vi "M5StackDAC2.vi"() -> ()   [LabVIEW 2024]
uses:
  Driver/Public/Digital Pull Direction.ctl
  4d20a38f-85d9-49a3-8b57-4ea18b2081fb.vi
  31698fb6-f1eb-4e5e-bade-b2e1298fca87.vi
  Driver/CTIPicoVISA.lvlib
panel:
  out "error out":errorcluster
  out "appended array":u8[](array[numeric])=[2, 208, 7, 7, 209] format="%.0x"
  in  "V1":u16(slide)=2001 scale=0.0..32767.0
  in  "V0":u16(slide)=2000 scale=0.0..32767.0
  in  "Grove Connector":enum16{"I2C0", "I2C1"}(ring)
  in  "VISA resource name in":refnum<visa-resource-name>="COM19"
  out "Identity":T1
  # "https://docs.m5stack.com/en/unit/Unit-DAC2"
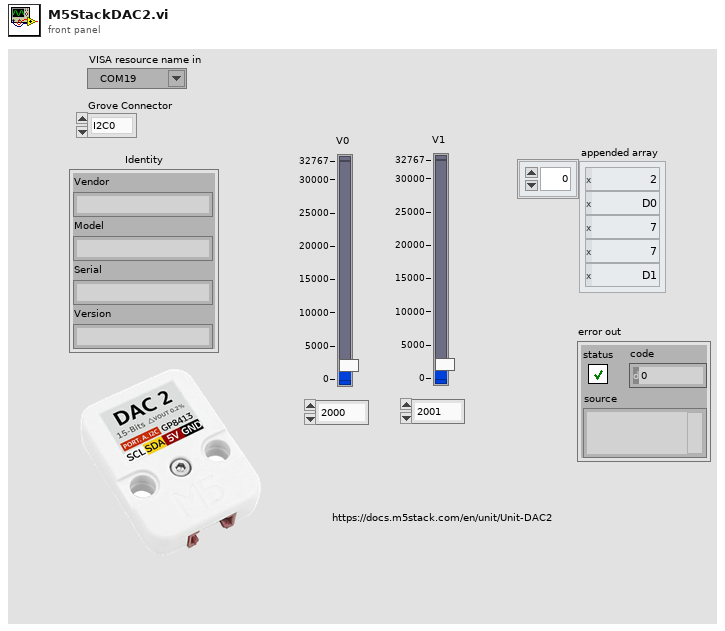
[diagram p1: front panel]
types:
  T1 = cluster{"Vendor":string, "Model":string, "Serial":string, "Version":string}
  T2 = typedef "CTIPicoVISA.lvlib/Digital Pull Direction.ctl" = enum16{"None", "Up", "Down", "Both"}
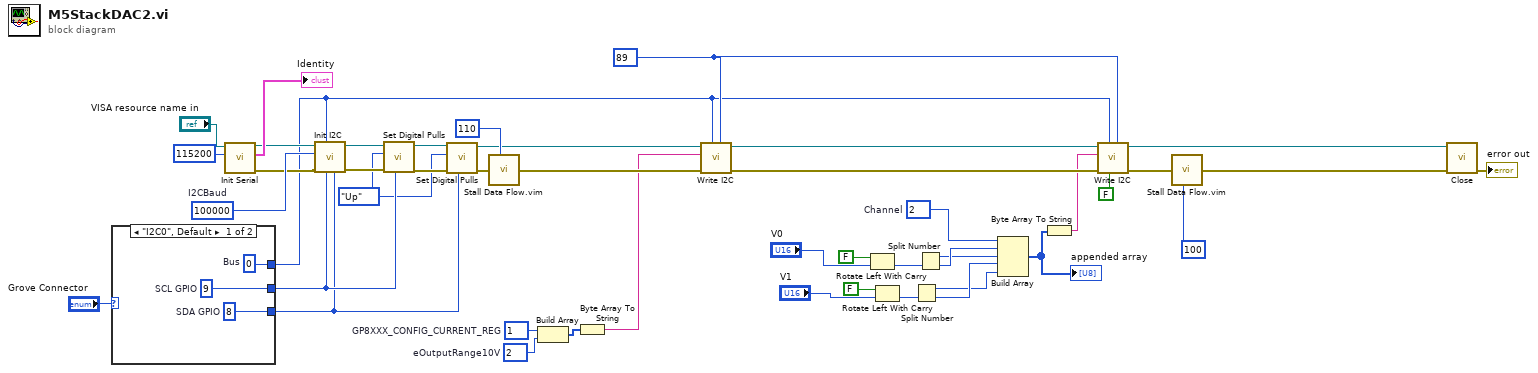
[diagram p0: block diagram]
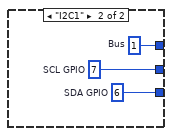
[diagram p2: hidden frame]
diagram:
  w12 = u8 2  # Channel
  w18 = u8 2  # eOutputRange10V
  w34 = Digital_Pull_Direction."Up" ("Pull")
  w41 = u32 100000  # I2CBaud
  w45 = u8 1  # GP8XXX_CONFIG_CURRENT_REG
  w22 = u8 89 ("Address")
  n1 = case shown="\"I2C0\", Default" "Grove Connector" {
    tunnel: [w48 w51] -> w35
    tunnel: [w47 w50] -> w33
    tunnel: [w46 w49] -> w19
    frame "I2C0", Default {
      w46 = u8 0  # Bus
      w47 = 8  # SDA GPIO
      w48 = 9  # SCL GPIO
    }
    frame "I2C1" {
      w49 = u8 1  # Bus
      w50 = 6  # SDA GPIO
      w51 = 7  # SCL GPIO
    }
  }
  n2 = call "Init Serial.vi"("Baud (115200)"=u32 115200, "VISA resource name in"="VISA resource name in") -> ("error out"=w29:errorcluster, "Identity"=→"Identity":T1, "VISA resource name Out"=w30:refnum<visa-resource-name>)  [unwired: 7 in]
  n3 = call "Init I2C.vi"("SDA GPIO"=w33, "SCL GPIO"=w35, "Bus"=w19, "error in (no error)"=w29, "Baud"=w41, "VISA resource name in"=w30) -> ("error out"=w38:errorcluster, "VISA resource name"=w39:refnum<visa-resource-name>)  [unwired: 4 in]
  n4 = call "Set Digital Pulls.vi"("GPIO"=w35, "error in (no error)"=w38, "Pull"=w34, "VISA resource name in"=w39) -> ("error out"=w36:errorcluster, "VISA resource name"=w37:refnum<visa-resource-name>)  [unwired: 6 in]
  n5 = call "Set Digital Pulls.vi"("GPIO"=w33, "error in (no error)"=w36, "Pull"=w34, "VISA resource name in"=w37) -> ("error out"=w31:errorcluster, "VISA resource name"=w25:refnum<visa-resource-name>)  [unwired: 6 in]
  n6 = call "Stall Data Flow.vim"("value in"=w31, "milliseconds to wait"=u32 110) -> ("value out"=w24:errorcluster)  [unwired: 1 out]
  n7 = Build Array(w45, w18) -> (w44:u8[])
  n8 = Byte Array To String(unsigned byte array=w44) -> (string=w23:string)
  n9 = call "Write I2C.vi"("Address"=w22, "Bus"=w19, "error in (no error)"=w24, "Data"=w23, "VISA resource name in"=w25) -> ("error out"=w20:errorcluster, "VISA resource name"=w21:refnum<visa-resource-name>)  [unwired: 5 in]
  n10 = Rotate Left With Carry(2:"V0", 3:FALSE ("carry")) -> (0:w9:u16)  [unwired: 1 out]
  n11 = Rotate Left With Carry(2:"V1", 3:FALSE ("carry")) -> (0:w7:u16)  [unwired: 1 out]
  n12 = Split Number(x=w7) -> (hi(x)=w1:u8, lo(x)=w2:u8)
  n13 = Split Number(x=w9) -> (hi(x)=w4:u8, lo(x)=w5:u8)
  n14 = Build Array(w12, w5, w4, w2, w1) -> (w13:u8[])
  "appended array" <- w13
  n15 = Byte Array To String(unsigned byte array=w13) -> (string=w16:string)
  n16 = call "Write I2C.vi"("Address"=w22, "NoStop (F)"=FALSE, "Bus"=w19, "error in (no error)"=w20, "Data"=w16, "VISA resource name in"=w21) -> ("error out"=w15:errorcluster, "VISA resource name"=w28:refnum<visa-resource-name>)  [unwired: 4 in]
  n17 = call "Stall Data Flow.vim"("value in"=w15, "milliseconds to wait"=u32 100) -> ("value out"=w27:errorcluster)  [unwired: 1 out]
  n18 = call "Close.vi"("error in (no error)"=w27, "VISA resource name in"=w28) -> ("error out"=→"error out":errorcluster)  [unwired: 9 in]
